vi "Disconnect.vi"(8 "Error In":errorcluster, 11 "Arduino Port":refnum<visa-resource-name>) -> (0 "Error Out":errorcluster)   [LabVIEW 2016]
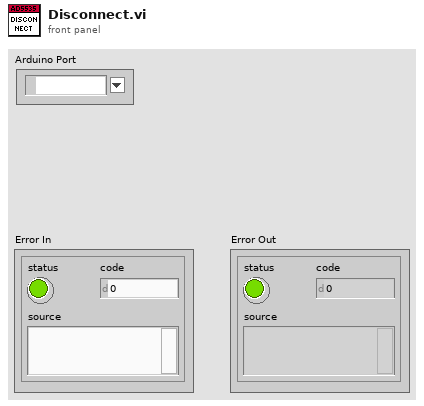
[diagram p1: front panel]
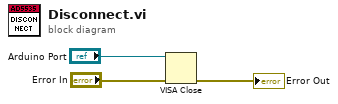
[diagram p0: block diagram]
diagram:
  n1 = VISA Close(VISA resource name="Arduino Port", error in (no error)="Error In") -> (error out=→"Error Out":errorcluster)
